vi "Auto Control.vi"   [LabVIEW 2018]
uses:
  <vilib>/Rock Robotics/Network Tables/NT Write String Array.vi
  SubSystems/Drive Train/Drive Train Global.vi
  Robot Global Data.vi
  SubSystems/Hatch Panel Intake/Hatch Panel Intake Global.vi
  SubSystems/Lift/Lift Global.vi
  SubSystems/Cargo Intake/Cargo Intake Global.vi
types:
  T1 = cluster{"X PID":cluster{"proportional gain (Kc)":dbl, "integral time (Ti, min)":dbl, "derivative time (Td, min)":dbl}, "Y PID":cluster{"proportional gain (Kc)":dbl, "integral time (Ti, min)":dbl, "derivative time (Td, min)":dbl}, "Z PID":cluster{"proportional gain (Kc)":dbl, "integral time (Ti, min)":dbl, "derivative time (Td, min)":dbl}}
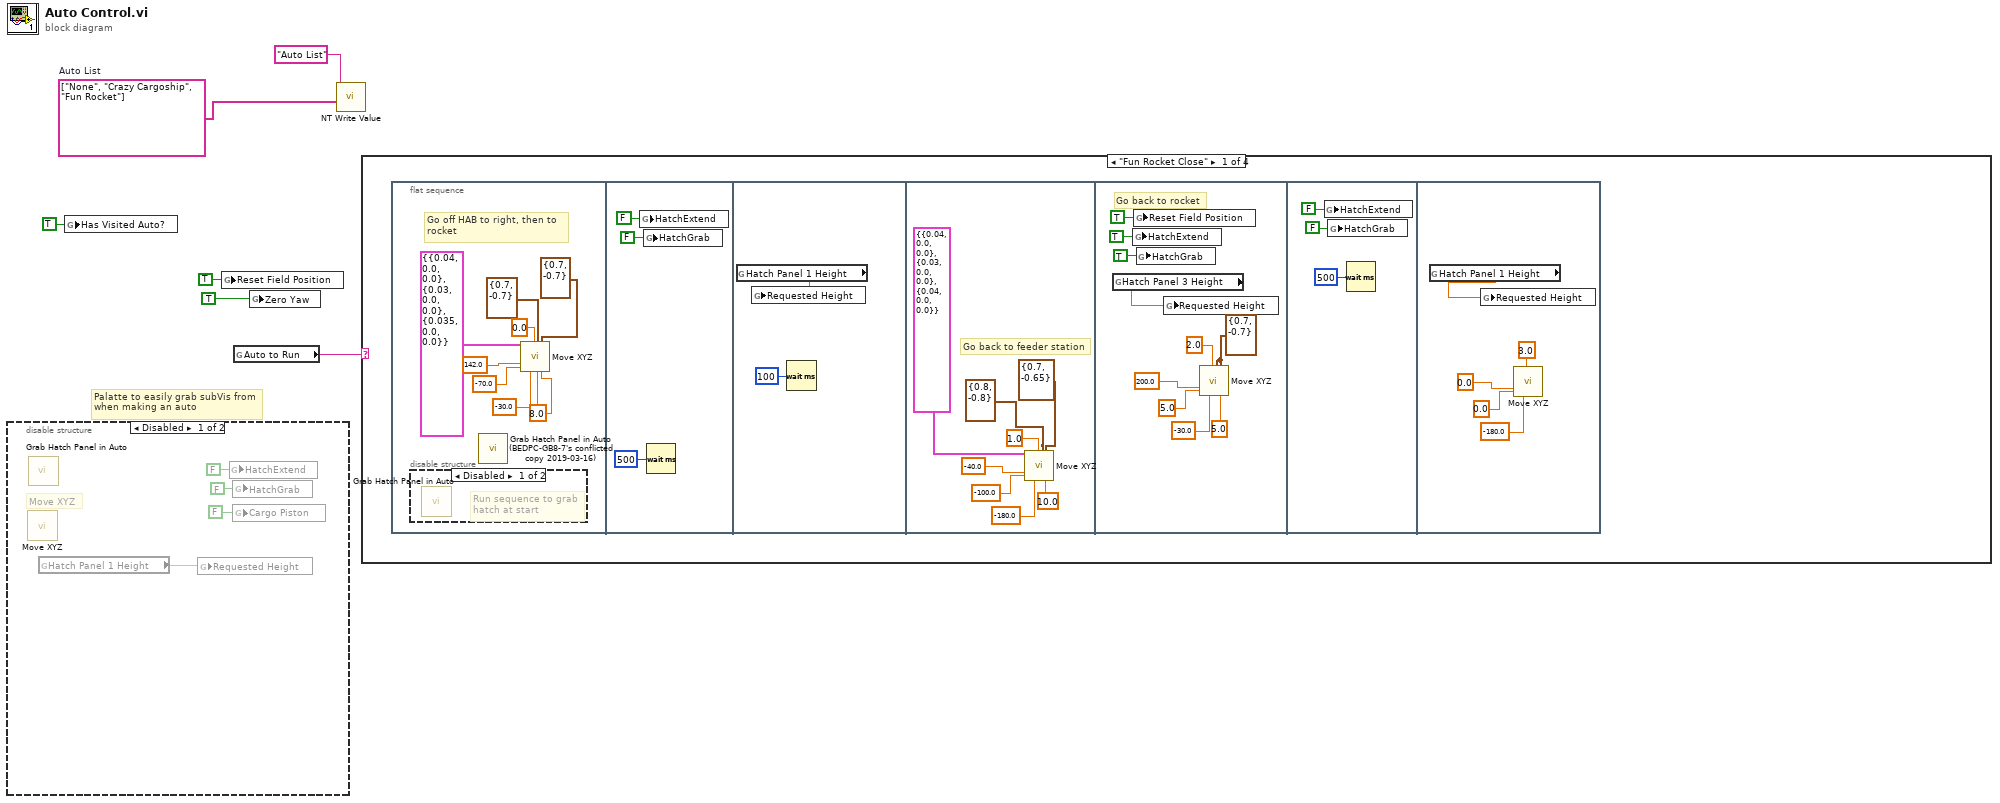
[diagram p0: block diagram]
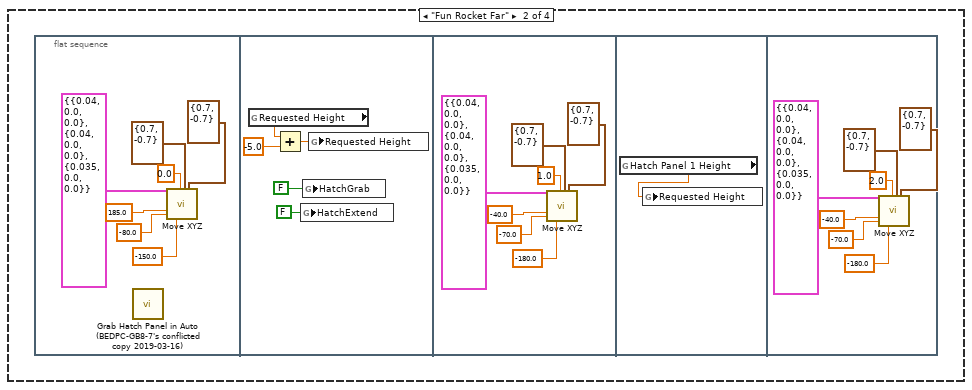
[diagram p4: hidden frame]
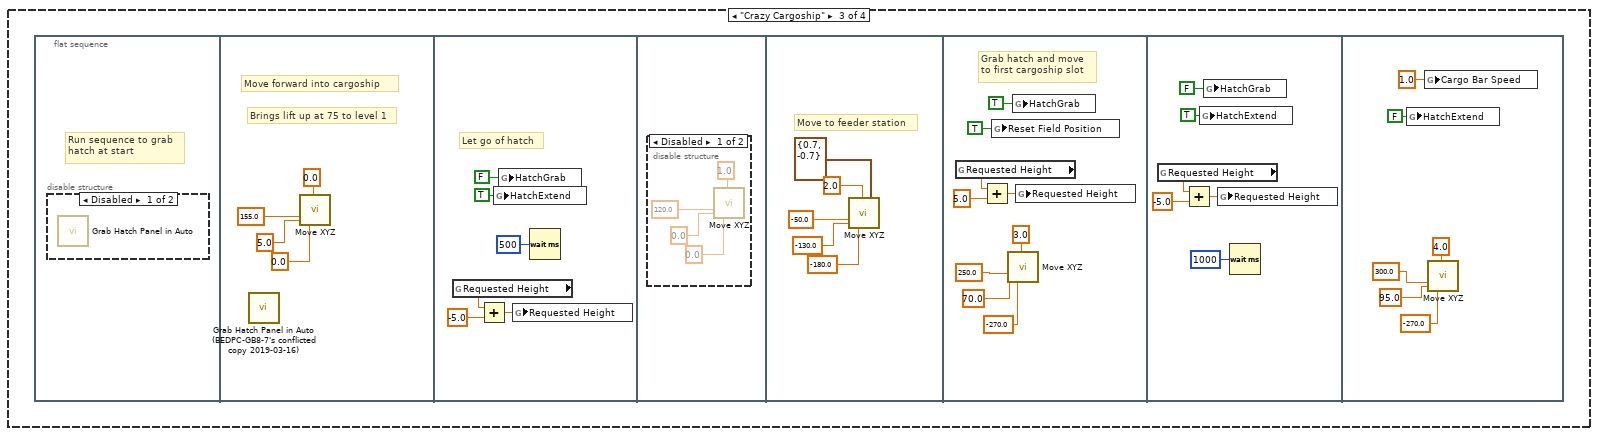
[diagram p5: hidden frame]
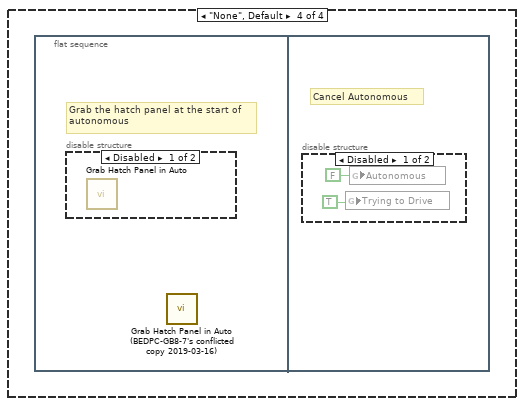
[diagram p8: hidden frame]
diagram:
  w5 = string[] ["None", "Crazy Cargoship", "Fun Rocket"]  # Auto List
  # "Palatte to easily grab subVis from\nwhen making an auto"
  n1 = disable-structure shown="Disabled" {
    frame Disabled {
      # "Move XYZ"
      n2 = call "Move XYZ.vi"() -> ()  [unwired: 28 in]
      n3 = call "Grab Hatch Panel in Auto.vi"() -> ()  [unwired: 12 in]
      n4 = global read "Lift Global.vi" "Hatch Panel 1 Height"() -> (w10:dbl)
      n5 = global write "Lift Global.vi" "Requested Height"(w10) -> ()
      n6 = global write "Hatch Panel Intake Global.vi" "HatchExtend"(FALSE ("HatchExtend")) -> ()
      n7 = global write "Hatch Panel Intake Global.vi" "HatchGrab"(FALSE ("HatchGrab")) -> ()
      n8 = global write "Cargo Intake Global.vi" "Cargo Piston"(FALSE ("Cargo Piston")) -> ()
    }
    frame Enabled {
    }
  }
  n9 = global write "Robot Global Data.vi" "Has Visited Auto?"(TRUE ("Has Visited Auto?")) -> ()
  n10 = global write "Drive Train Global.vi" "Reset Field Position"(TRUE ("Reset Field Position")) -> ()
  n11 = global read "Robot Global Data.vi" "Auto to Run"() -> (w4:string)
  n12 = global write "Drive Train Global.vi" "Zero Yaw"(TRUE ("Reset Field Position")) -> ()
  n13 = call-poly <vilib>:"NT Write Value.vi"("String Array"=w5, "Name"="Auto List") -> ()  [unwired: 9 in, 1 out]
  n14 = case shown="\"Fun Rocket Close\"" w4 {
    frame "Fun Rocket Close" {
      n15 = flat-sequence {
        frame #0 {
          w12 = 8.0 ("X Stop Threshold")
          # "Go off HAB to right, then to\nrocket"
          n16 = disable-structure shown="Disabled" {
            frame Disabled {
              # "Run sequence to grab\nhatch at start"
              n17 = call "Grab Hatch Panel in Auto.vi"() -> ()  [unwired: 12 in]
            }
            frame Enabled {
            }
          }
          n18 = call "Grab Hatch Panel in Auto (BEDPC-GB8-7's conflicted copy 2019-03-16).vi"() -> ()  [unwired: 12 in]
          n19 = call "Move XYZ.vi"("PID Gains In"=T1 {"X PID"={"proportional gain (Kc)"=0.04, "integral time (Ti, min)"=0.0, "derivative time (Td, min)"=0.0}, "Y PID"={"proportional gain (Kc)"=0.03, "integral time (Ti, min)"=0.0, "derivative time (Td, min)"=0.0}, "Z PID"={"proportional gain (Kc)"=0.035, "integral time (Ti, min)"=0.0, "derivative time (Td, min)"=0.0}}, "Y Target"=142.0, "X Target"=-70.0, "Gyro Target"=-30.0, "Movement"=0.0, "X Output Range"=cluster{"output high":dbl, "output low":dbl} {"output high"=0.7, "output low"=-0.7}, "X Stop Threshold"=w12, "Y Output Range"=cluster{"output high":dbl, "output low":dbl} {"output high"=0.7, "output low"=-0.7} ("X Output Range"), "Y Stop Threshold"=w12) -> ()  [unwired: 19 in]
        }
        frame #1 {
          n20 = global write "Hatch Panel Intake Global.vi" "HatchExtend"(FALSE ("HatchExtend")) -> ()
          n21 = global write "Hatch Panel Intake Global.vi" "HatchGrab"(FALSE ("HatchGrab")) -> ()
          n22 = Wait (ms)(milliseconds to wait=u32 500) -> ()  [unwired: 1 out]
        }
        frame #2 {
          n23 = global read "Lift Global.vi" "Hatch Panel 1 Height"() -> (w23:dbl)
          n24 = global write "Lift Global.vi" "Requested Height"(w23) -> ()
          n25 = Wait (ms)(milliseconds to wait=u32 100) -> ()  [unwired: 1 out]
        }
        frame #3 {
          # "Go back to feeder station"
          n26 = call "Move XYZ.vi"("PID Gains In"=T1 {"X PID"={"proportional gain (Kc)"=0.04, "integral time (Ti, min)"=0.0, "derivative time (Td, min)"=0.0}, "Y PID"={"proportional gain (Kc)"=0.03, "integral time (Ti, min)"=0.0, "derivative time (Td, min)"=0.0}, "Z PID"={"proportional gain (Kc)"=0.04, "integral time (Ti, min)"=0.0, "derivative time (Td, min)"=0.0}}, "Y Target"=-40.0, "X Target"=-100.0, "Gyro Target"=-180.0, "Movement"=1.0, "X Output Range"=cluster{"output high":dbl, "output low":dbl} {"output high"=0.8, "output low"=-0.8}, "Y Output Range"=cluster{"output high":dbl, "output low":dbl} {"output high"=0.7, "output low"=-0.65} ("X Output Range"), "Y Stop Threshold"=10.0) -> ()  [unwired: 20 in]
        }
        frame #4 {
          w32 = cluster{"output high":dbl, "output low":dbl} {"output high"=0.7, "output low"=-0.7} ("Y Output Range")
          # "Go back to rocket"
          n27 = global read "Lift Global.vi" "Hatch Panel 3 Height"() -> (w34:dbl)
          n28 = global write "Hatch Panel Intake Global.vi" "HatchExtend"(TRUE ("HatchExtend")) -> ()
          n29 = global write "Drive Train Global.vi" "Reset Field Position"(TRUE ("Reset Field Position")) -> ()
          n30 = global write "Hatch Panel Intake Global.vi" "HatchGrab"(TRUE ("HatchGrab")) -> ()
          n31 = global write "Lift Global.vi" "Requested Height"(w34) -> ()
          n32 = call "Move XYZ.vi"("Y Target"=200.0, "X Target"=5.0, "Gyro Target"=-30.0, "Movement"=2.0, "X Output Range"=w32, "Y Output Range"=w32, "Y Stop Threshold"=5.0) -> ()  [unwired: 21 in]
        }
        frame #5 {
          n33 = global write "Hatch Panel Intake Global.vi" "HatchExtend"(FALSE ("HatchExtend")) -> ()
          n34 = global write "Hatch Panel Intake Global.vi" "HatchGrab"(FALSE ("HatchGrab")) -> ()
          n35 = Wait (ms)(milliseconds to wait=u32 500) -> ()  [unwired: 1 out]
        }
        frame #6 {
          n36 = global read "Lift Global.vi" "Hatch Panel 1 Height"() -> (w49:dbl)
          n37 = global write "Lift Global.vi" "Requested Height"(w49) -> ()
          n38 = call "Move XYZ.vi"("Y Target"=0.0, "X Target"=0.0, "Gyro Target"=-180.0, "Movement"=3.0) -> ()  [unwired: 24 in]
        }
      }
    }
    frame "Fun Rocket Far" {
      n39 = flat-sequence {
        frame #0 {
          n40 = call "Grab Hatch Panel in Auto (BEDPC-GB8-7's conflicted copy 2019-03-16).vi"() -> ()  [unwired: 12 in]
          n41 = call "Move XYZ.vi"("PID Gains In"=T1 {"X PID"={"proportional gain (Kc)"=0.04, "integral time (Ti, min)"=0.0, "derivative time (Td, min)"=0.0}, "Y PID"={"proportional gain (Kc)"=0.04, "integral time (Ti, min)"=0.0, "derivative time (Td, min)"=0.0}, "Z PID"={"proportional gain (Kc)"=0.035, "integral time (Ti, min)"=0.0, "derivative time (Td, min)"=0.0}}, "Y Target"=185.0, "X Target"=-80.0, "Gyro Target"=-150.0, "Movement"=0.0, "X Output Range"=cluster{"output high":dbl, "output low":dbl} {"output high"=0.7, "output low"=-0.7}, "Y Output Range"=cluster{"output high":dbl, "output low":dbl} {"output high"=0.7, "output low"=-0.7} ("X Output Range")) -> ()  [unwired: 21 in]
        }
        frame #1 {
          n42 = global read "Lift Global.vi" "Requested Height"() -> (w58:dbl)
          n43 = Add(x=w58, y=-5.0) -> (x+y=w57:dbl)
          n44 = global write "Hatch Panel Intake Global.vi" "HatchExtend"(FALSE ("HatchExtend")) -> ()
          n45 = global write "Hatch Panel Intake Global.vi" "HatchGrab"(FALSE ("HatchExtend")) -> ()
          n46 = global write "Lift Global.vi" "Requested Height"(w57) -> ()
        }
        frame #2 {
          n47 = call "Move XYZ.vi"("PID Gains In"=T1 {"X PID"={"proportional gain (Kc)"=0.04, "integral time (Ti, min)"=0.0, "derivative time (Td, min)"=0.0}, "Y PID"={"proportional gain (Kc)"=0.04, "integral time (Ti, min)"=0.0, "derivative time (Td, min)"=0.0}, "Z PID"={"proportional gain (Kc)"=0.035, "integral time (Ti, min)"=0.0, "derivative time (Td, min)"=0.0}}, "Y Target"=-40.0, "X Target"=-70.0, "Gyro Target"=-180.0, "Movement"=1.0, "X Output Range"=cluster{"output high":dbl, "output low":dbl} {"output high"=0.7, "output low"=-0.7}, "Y Output Range"=cluster{"output high":dbl, "output low":dbl} {"output high"=0.7, "output low"=-0.7} ("X Output Range")) -> ()  [unwired: 21 in]
        }
        frame #3 {
          n48 = global read "Lift Global.vi" "Hatch Panel 1 Height"() -> (w69:dbl)
          n49 = global write "Lift Global.vi" "Requested Height"(w69) -> ()
        }
        frame #4 {
          n50 = call "Move XYZ.vi"("PID Gains In"=T1 {"X PID"={"proportional gain (Kc)"=0.04, "integral time (Ti, min)"=0.0, "derivative time (Td, min)"=0.0}, "Y PID"={"proportional gain (Kc)"=0.04, "integral time (Ti, min)"=0.0, "derivative time (Td, min)"=0.0}, "Z PID"={"proportional gain (Kc)"=0.035, "integral time (Ti, min)"=0.0, "derivative time (Td, min)"=0.0}}, "Y Target"=-40.0, "X Target"=-70.0, "Gyro Target"=-180.0, "Movement"=2.0, "X Output Range"=cluster{"output high":dbl, "output low":dbl} {"output high"=0.7, "output low"=-0.7}, "Y Output Range"=cluster{"output high":dbl, "output low":dbl} {"output high"=0.7, "output low"=-0.7} ("X Output Range")) -> ()  [unwired: 21 in]
        }
      }
    }
    frame "Crazy Cargoship" {
      n51 = flat-sequence {
        frame #0 {
          # "Run sequence to grab\nhatch at start"
          n52 = disable-structure shown="Disabled" {
            frame Disabled {
              n53 = call "Grab Hatch Panel in Auto.vi"() -> ()  [unwired: 12 in]
            }
            frame Enabled {
            }
          }
        }
        frame #1 {
          # "Brings lift up at 75 to level 1"
          # "Move forward into cargoship"
          n54 = call "Grab Hatch Panel in Auto (BEDPC-GB8-7's conflicted copy 2019-03-16).vi"() -> ()  [unwired: 12 in]
          n55 = call "Move XYZ.vi"("Y Target"=155.0, "X Target"=5.0, "Gyro Target"=0.0, "Movement"=0.0) -> ()  [unwired: 24 in]
        }
        frame #2 {
          # "Let go of hatch"
          n56 = global read "Lift Global.vi" "Requested Height"() -> (w82:dbl)
          n57 = Add(x=w82, y=-5.0) -> (x+y=w81:dbl)
          n58 = global write "Hatch Panel Intake Global.vi" "HatchExtend"(TRUE ("HatchGrab")) -> ()
          n59 = global write "Hatch Panel Intake Global.vi" "HatchGrab"(FALSE ("HatchGrab")) -> ()
          n60 = global write "Lift Global.vi" "Requested Height"(w81) -> ()
          n61 = Wait (ms)(milliseconds to wait=u32 500) -> ()  [unwired: 1 out]
        }
        frame #3 {
          n62 = disable-structure shown="Disabled" {
            frame Disabled {
              n63 = call "Move XYZ.vi"("Y Target"=120.0, "X Target"=0.0, "Gyro Target"=0.0, "Movement"=1.0) -> ()  [unwired: 24 in]
            }
            frame Enabled {
            }
          }
        }
        frame #4 {
          # "Move to feeder station"
          n64 = call "Move XYZ.vi"("Y Target"=-50.0, "X Target"=-130.0, "Gyro Target"=-180.0, "Movement"=2.0, "Y Output Range"=cluster{"output high":dbl, "output low":dbl} {"output high"=0.7, "output low"=-0.7}) -> ()  [unwired: 23 in]
        }
        frame #5 {
          # "Grab hatch and move\nto first cargoship slot"
          n65 = global read "Lift Global.vi" "Requested Height"() -> (w100:dbl)
          n66 = Add(x=w100, y=5.0) -> (x+y=w101:dbl)
          n67 = global write "Drive Train Global.vi" "Reset Field Position"(TRUE ("Reset Field Position")) -> ()
          n68 = call "Move XYZ.vi"("Y Target"=250.0, "X Target"=70.0, "Gyro Target"=-270.0, "Movement"=3.0) -> ()  [unwired: 24 in]
          n69 = global write "Hatch Panel Intake Global.vi" "HatchGrab"(TRUE ("HatchGrab")) -> ()
          n70 = global write "Lift Global.vi" "Requested Height"(w101) -> ()
        }
        frame #6 {
          n71 = global read "Lift Global.vi" "Requested Height"() -> (w107:dbl)
          n72 = Add(x=w107, y=-5.0) -> (x+y=w106:dbl)
          n73 = global write "Hatch Panel Intake Global.vi" "HatchExtend"(TRUE ("HatchGrab")) -> ()
          n74 = global write "Hatch Panel Intake Global.vi" "HatchGrab"(FALSE ("HatchGrab")) -> ()
          n75 = global write "Lift Global.vi" "Requested Height"(w106) -> ()
          n76 = Wait (ms)(milliseconds to wait=u32 1000) -> ()  [unwired: 1 out]
        }
        frame #7 {
          n77 = global write "Hatch Panel Intake Global.vi" "HatchExtend"(FALSE ("HatchGrab")) -> ()
          n78 = global write "Cargo Intake Global.vi" "Cargo Bar Speed"(1.0 ("Cargo Bar Speed")) -> ()
          n79 = call "Move XYZ.vi"("Y Target"=300.0, "X Target"=95.0, "Gyro Target"=-270.0, "Movement"=4.0) -> ()  [unwired: 24 in]
        }
      }
    }
    frame "None", Default {
      n80 = flat-sequence {
        frame #0 {
          # "Grab the hatch panel at the start of \nautonomous"
          n81 = disable-structure shown="Disabled" {
            frame Disabled {
              n82 = call "Grab Hatch Panel in Auto.vi"() -> ()  [unwired: 12 in]
            }
            frame Enabled {
            }
          }
          n83 = call "Grab Hatch Panel in Auto (BEDPC-GB8-7's conflicted copy 2019-03-16).vi"() -> ()  [unwired: 12 in]
        }
        frame #1 {
          # "Cancel Autonomous"
          n84 = disable-structure shown="Disabled" {
            frame Disabled {
              n85 = global write "Robot Global Data.vi" "Trying to Drive"(TRUE ("Autonomous")) -> ()
              n86 = global write "Robot Global Data.vi" "Autonomous"(FALSE ("Autonomous")) -> ()
            }
            frame Enabled {
            }
          }
        }
      }
    }
  }
